vi "Que step.vi"() -> (13 "Que name":string="Main")   [LabVIEW 2014, in "Que lib.lvlib"]
uses:
  Que lib.lvlib
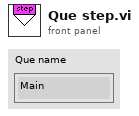
[diagram p1: front panel]
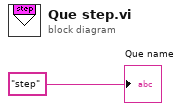
[diagram p0: block diagram]
diagram:
  "Que name" <- "step"
